vi "Initialize Stablizing Display.vi"(8 "error in (no error)":errorcluster, 11 "output cluster":T1) -> (0 "error out":errorcluster, 3 "Array":dbl[](array[numeric]))   [LabVIEW 2016]
uses:
  Controls/Cal Refs.ctl
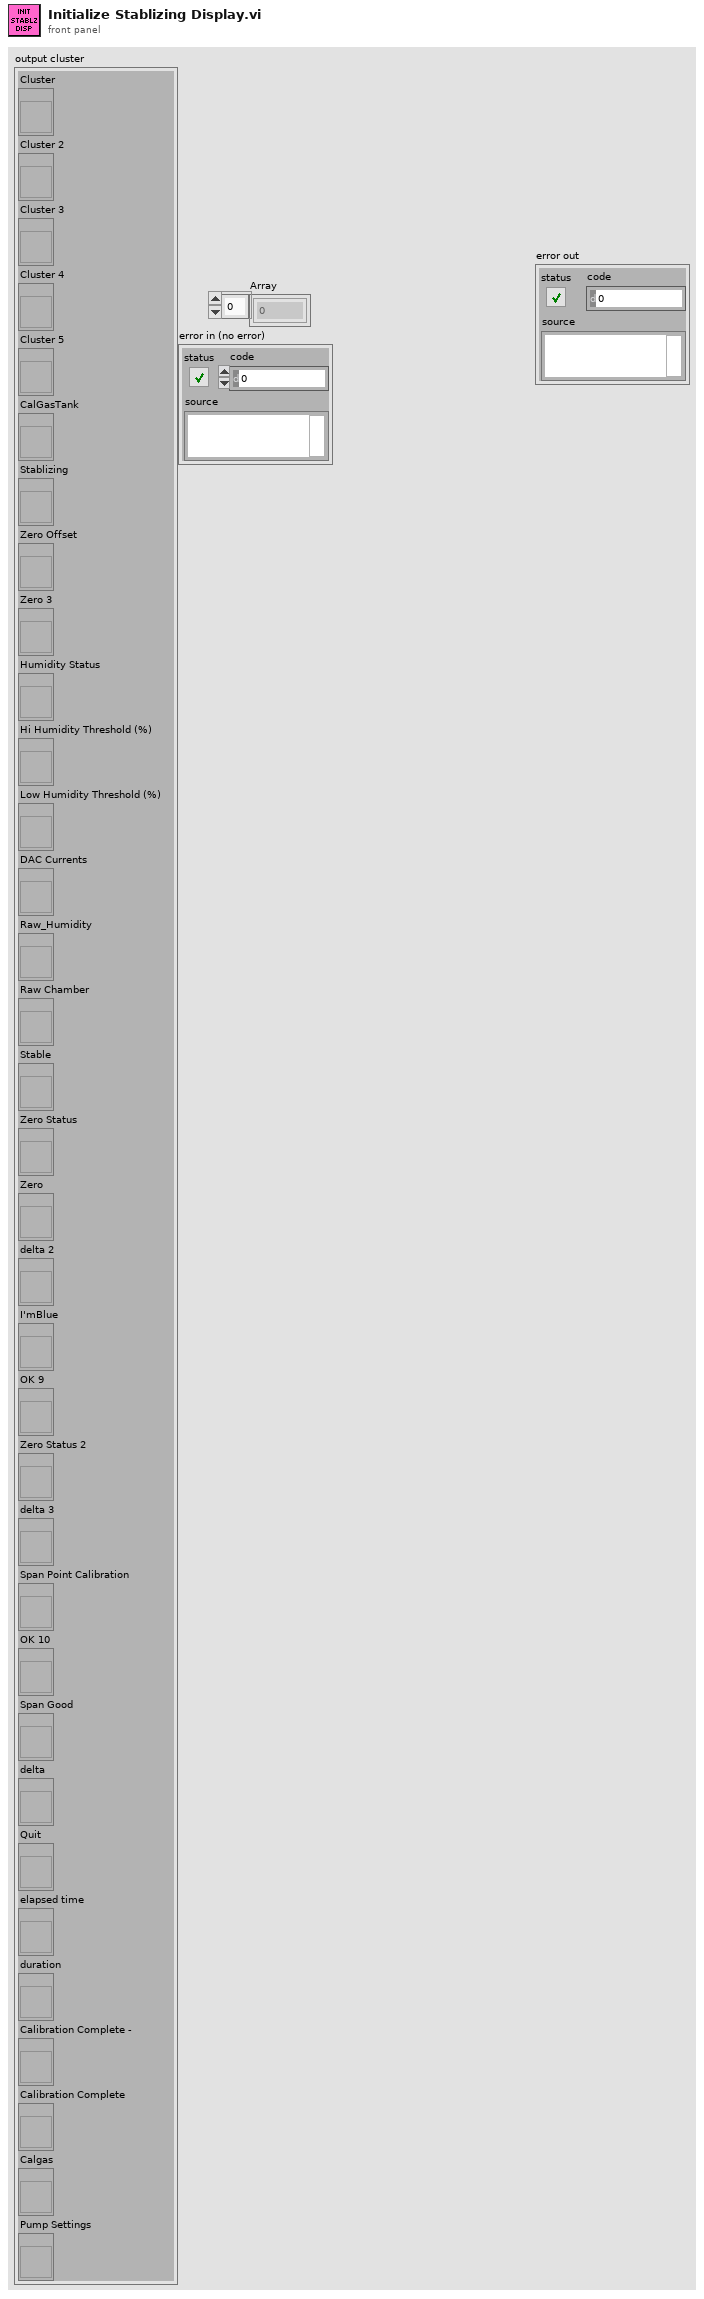
[diagram p1: front panel]
types:
  T1 = typedef "Cal Refs.ctl" = cluster{"Cluster":refnum<vi>, "Cluster 2":refnum<vi>, "Cluster 3":refnum<vi>, "Cluster 4":refnum<vi>, "Cluster 5":refnum<vi>, "CalGasTank":refnum<vi>, "Stablizing":refnum<vi>, "Zero Offset":refnum<vi>, "Zero 3":refnum<vi>, "Humidity Status":refnum<vi>, "Hi Humidity Threshold (%)":refnum<vi>, "Low Humidity Threshold (%)":refnum<vi>, "DAC Currents":refnum<vi>, "Raw_Humidity":refnum<vi>, "Raw Chamber":refnum<vi>, "Stable":refnum<vi>, "Zero Status":refnum<vi>, "Zero":refnum<vi>, "delta 2":refnum<vi>, "I'mBlue":refnum<vi>, "OK 9":refnum<vi>, "Zero Status 2":refnum<vi>, "delta 3":refnum<vi>, "Span Point Calibration":refnum<vi>, "OK 10":refnum<vi>, "Span Good":refnum<vi>, "delta":refnum<vi>, "Quit":refnum<vi>, "elapsed time":refnum<vi>, "duration":refnum<vi>, "Calibration Complete -":refnum<vi>, "Calibration Complete":refnum<vi>, "Calgas":refnum<vi>, "Pump Settings":refnum<vi>}
  T2 = enum16{"Waiting For Film to Stabilize", "Film Stable", "Exiting", "Initializing"}
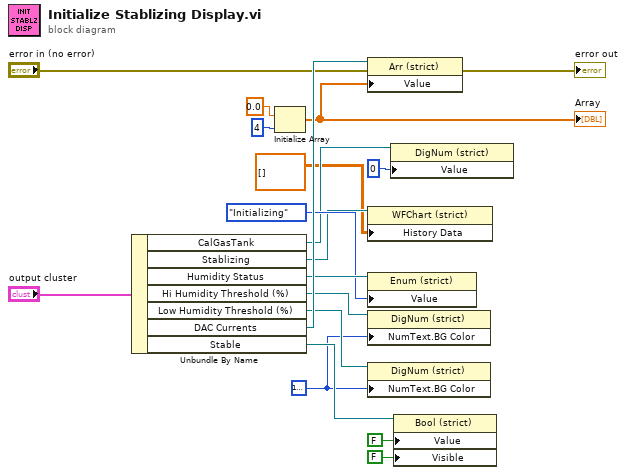
[diagram p0: block diagram]
diagram:
  w4 = u32 16777216
  n1 = Unbundle By Name("output cluster") -> ("CalGasTank"=w9:refnum<vi>, "Stablizing"=w8:refnum<vi>, "Humidity Status"=w14:refnum<vi>, "Hi Humidity Threshold (%)"=w15:refnum<vi>, "Low Humidity Threshold (%)"=w16:refnum<vi>, "DAC Currents"=w17:refnum<vi>, "Stable"=w18:refnum<vi>)
  n2 = Initialize Array(0.0, 4 ("dimension size")) -> (w13:dbl[])
  "Array" <- w13
  n3 = property class="Arr (strict)"(reference=w17, error in="error in (no error)", "Value"=w13) -> (error out=→"error out":errorcluster)  [unwired: 1 out]
  n4 = property on="Property Node" class="WFChart (strict)"(reference=w8, "History Data"=dbl[][] []) -> ()  [unwired: 1 in, 2 out]
  n5 = property class="Enum (strict)"(reference=w14, "Value"=T2."Initializing" ("Humidity Status")) -> ()  [unwired: 1 in, 2 out]
  n6 = property on="Property Node" class="DigNum (strict)"(reference=w15, "NumText.BG Color"=w4) -> ()  [unwired: 1 in, 2 out]
  n7 = property on="Property Node" class="DigNum (strict)"(reference=w16, "NumText.BG Color"=w4) -> ()  [unwired: 1 in, 2 out]
  n8 = property class="DigNum (strict)"(reference=w9, "Value"=u8 0 ("CalGasTank")) -> ()  [unwired: 1 in, 2 out]
  n9 = property on="Property Node" class="Bool (strict)"(reference=w18, "Value"=FALSE ("Done"), "Visible"=FALSE) -> ()  [unwired: 1 in, 2 out]
